vi "PrefDialog.vi"(8 "error in (no error)":errorcluster, 11 "MyPluginsBase in":refnum<class "ChromaAcLoad.lvclass">) -> (0 "error out":errorcluster, 1 "Save As":bool, 2 "Changed":bool, 3 "MyPluginsBase out":refnum<class "ChromaAcLoad.lvclass">)   [LabVIEW 2018, in "AcPwrPlugins.lvlib" / "ChromaAcLoad.lvclass"]
doc: "This VI opens up the modal preference dialog window and allows a user to configure the dialog with a new configuration or the existing configuration that was previously saved to file. The user can also chose to save the new configuration to the existing file location with the save boolean or a new file location by using the save as boolean."
uses:
  ChromaAcLoad.lvclass
  C:/Program Files (x86)/National Instruments/LabVIEW 2018/user.lib/NIST/BaseClasses/BasePlugin_class/BasePlugin.lvclass
  C:/Users/ico/Documents/Projects/NistPluggableModules/AcPwr/AcPwrPlugins/AcPwrBaseClass/AcPwrBase.lvclass
  TypeDefs/Load.ctl
  TypeDefs/LoadSettings.ctl
  TypeDefs/LC.ctl
  TypeDefs/LoadModes.ctl
  AcPwrBaseClass/TypeDefs/BaseMeasure.ctl
  AcPwrBaseClass/TypeDefs/MeasType.ctl
  AcPwrBaseClass/TypeDefs/BaseConfig.ctl
  AcPwrBaseClass/TypeDefs/Phase.ctl
  <userlib>/NIST/BaseClasses/BasePlugin_class/BasePlugin.lvclass/BasePlugin.ctl
  AcPwrBaseClass/AcPwrBase.lvclass/AcPwrBase.ctl
  ChromaAcLoad.lvclass/ChromaAcLoad.ctl
  <userlib>/NIST/BaseClasses/BasePlugin_class/Accessors/Read PluginIniFilePath.vi
  AcPwrBaseClass/Accessors/Read BaseConfig.vi
  Accessors/Read Loads.vi
  AcPwrBaseClass/Accessors/Read BaseMeasures.vi
  AcPwrBaseClass/Accessors/Read RefreshTime.vi
  AcPwrBaseClass/Accessors/Write BaseConfig.vi
  Accessors/Write Loads.vi
  AcPwrBaseClass/Accessors/Write BaseMeasures.vi
  AcPwrBaseClass/Accessors/Write RefreshTime.vi
  <vilib>/Utility/config.llb/NI_LVConfig.lvlib
  AcPwrBaseClass/AcPwrBase.lvclass
panel:
  in  "Load Numerical Configuration":T1(array[cluster])
  in  "Loads":T2(array[ring])
  in  "Slew Rate (Units/S)":T3
  in  "btnSaveAs":bool
  in  "BaseConfig":T4
  in  "RefreshTime":dbl
  in  "Measurements":T6[](array[typedef])
  in  "Loads":T8[](array[typedef])
  in  "btnSave":bool
  in  "btnCancel":bool
  # "AC is compatible with: CC, CR, CP, RLC, RLC CP, and Inrush\n\nDC is compatible with: CC, CR, CP, CV, and Rectified"
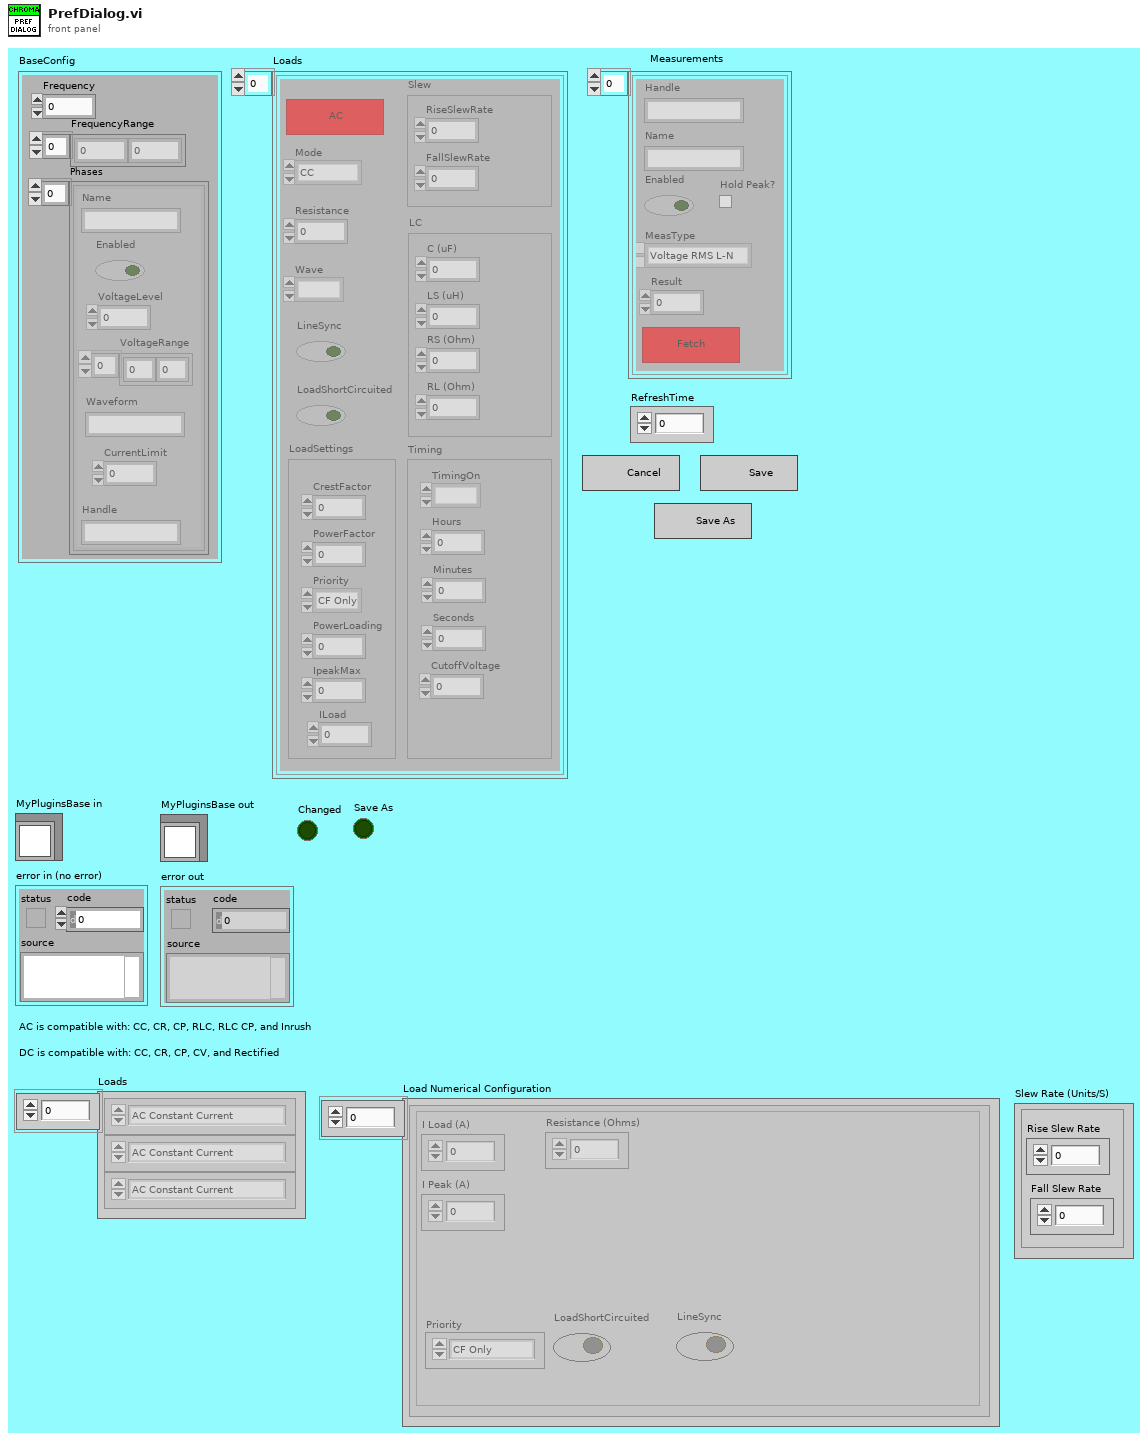
[diagram p1: front panel]
types:
  T1 = cluster{"I Load (A)":dbl, "I Peak (A)":dbl, "Resistance (Ohms)":dbl, "Priority":enum16{"CF Only", "PF Only", "Both (CF)", "Both (PF)"}, "LoadShortCircuited":bool, "LineSync":bool}[]
  T2 = enum16{"AC Constant Current", "AC Constant Resistance", "AC Constant Power", "AC RLC", "AC RL Constant Power", "AC Inrush", "DC Constant Current", "DC Constant Resistance", "DC Constant Power", "DC Constant Voltage", "DC Rectified"}[]
  T3 = cluster{"Rise Slew Rate":dbl, "Fall Slew Rate":dbl}
  T4 = typedef "AcPwrPlugins.lvlib/AcPwrBase.lvclass/BaseConfig.ctl" = cluster{"Frequency":dbl, "FrequencyRange":dbl[], "Phases":T5[]}
  T5 = typedef "AcPwrPlugins.lvlib/AcPwrBase.lvclass/Phase.ctl" = cluster{"Enabled":bool, "VoltageLevel":dbl, "Waveform":string, "Name":string, "VoltageRange":dbl[], "CurrentLimit":dbl, "Handle":string, "Connected":bool}
  T6 = typedef "AcPwrPlugins.lvlib/AcPwrBase.lvclass/BaseMeasure.ctl" = cluster{"Handle":string, "Name":string, "Enabled":bool, "Result":dbl, "MeasType":T7, "btnMeasFetch":bool, "Hold Peak?":bool}
  T7 = typedef "AcPwrPlugins.lvlib/AcPwrBase.lvclass/MeasType.ctl" = enum16{"Voltage RMS L-N", "Current RMS", "Frequency", "Voltage DC", "Current DC", "Power Factor", "Current Peak", "Power VA", "Real Power", "Voltage THD", "Voltage EHD", "Voltage OHD", "Current THD", "Current EHD", "Current OHD", "Voltage RMS L-L", "Phase Angle", "Power DC", "Crest Factor"}
  T8 = typedef "AcPwrPlugins.lvlib/ChromaAcLoad.lvclass/Load.ctl" = cluster{"AC/DC":bool, "Resistance":dbl, "LoadSettings":T9, "Wave":enum16{""}, "LineSync":bool, "LoadShortCircuited":bool, "LC":T10, "Timing":cluster{"TimingOn":enum16{""}, "Hours":u32, "Minutes":u32, "Seconds":dbl, "CutoffVoltage":dbl}, "Slew":cluster{"RiseSlewRate":i32, "FallSlewRate":i32}, "Mode":T11}
  T9 = typedef "AcPwrPlugins.lvlib/ChromaAcLoad.lvclass/LoadSettings.ctl" = cluster{"CrestFactor":dbl, "PowerFactor":dbl, "PowerLoading":dbl, "IpeakMax":dbl, "Priority":enum16{"CF Only", "PF Only", "Both (CF)", "Both (PF)"}, "ILoad":dbl}
  T10 = typedef "AcPwrPlugins.lvlib/ChromaAcLoad.lvclass/LC.ctl" = cluster{"C (uF)":i32, "LS (uH)":i32, "RL (Ohm)":dbl, "RS (Ohm)":dbl}
  T11 = typedef "AcPwrPlugins.lvlib/ChromaAcLoad.lvclass/LoadModes.ctl" = enum16{"CC", "CP", "CV", "CR", "RLC", "RLC CP", "Inrush", "Rectified"}
  T12 = enum8{"Enabled", "Disabled", "Disabled and Grayed Out"}
  T13 = enum32{"Invalid", "Default", "Floating", "Floating/Auto-Hide", "Modal"}
  T14 = enum32{"Invalid", "Standard", "Closed", "Hidden", "Minimized", "Maximized"}
  T15 = typedef "NI_LVConfig.lvlib/Config Data RefNum.ctl" = refnum<k1>
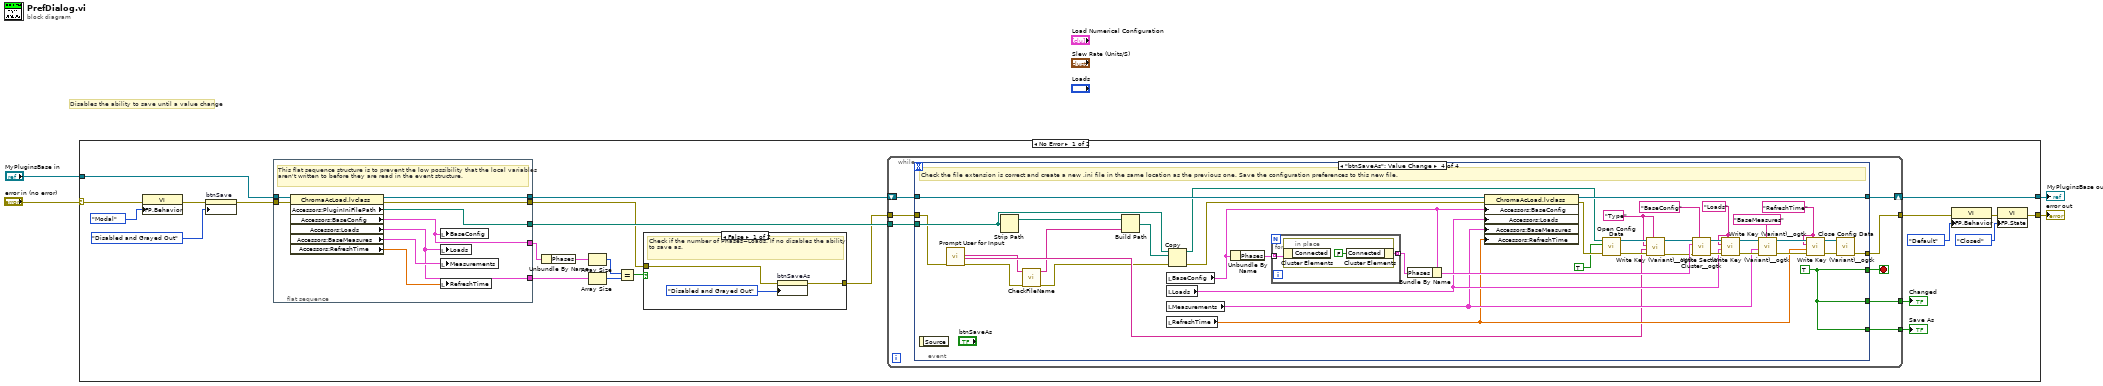
[diagram p0: block diagram]
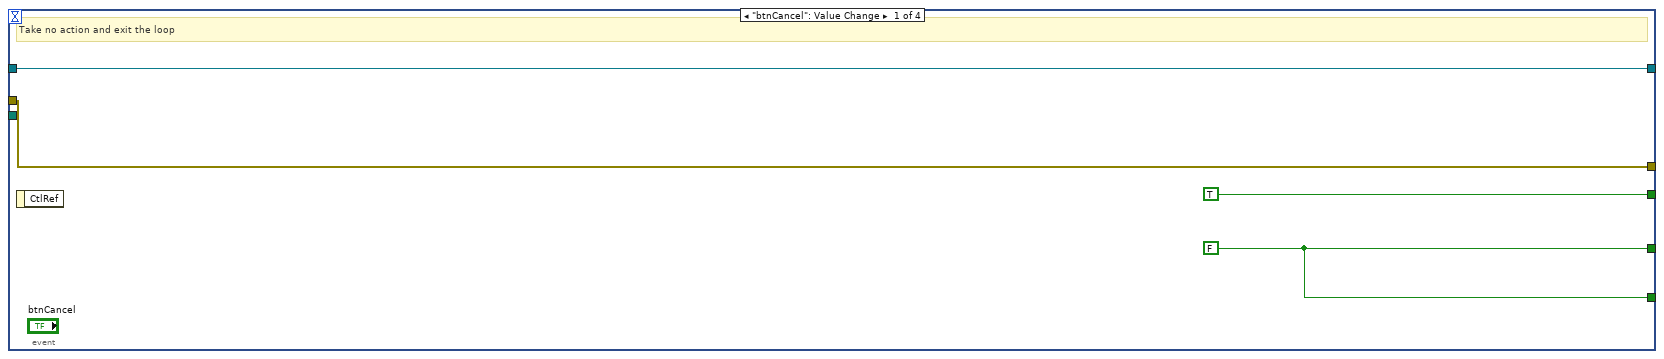
[diagram p3: hidden frame]
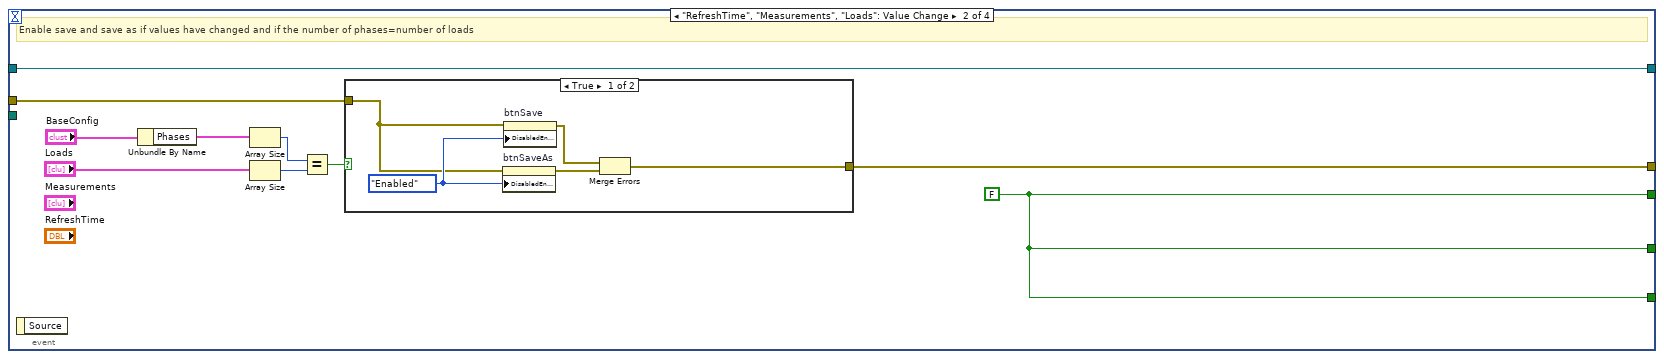
[diagram p4: hidden frame]
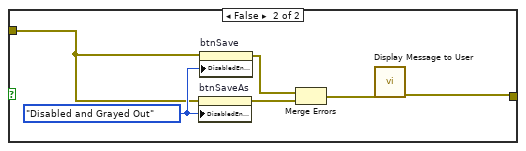
[diagram p5: hidden frame]
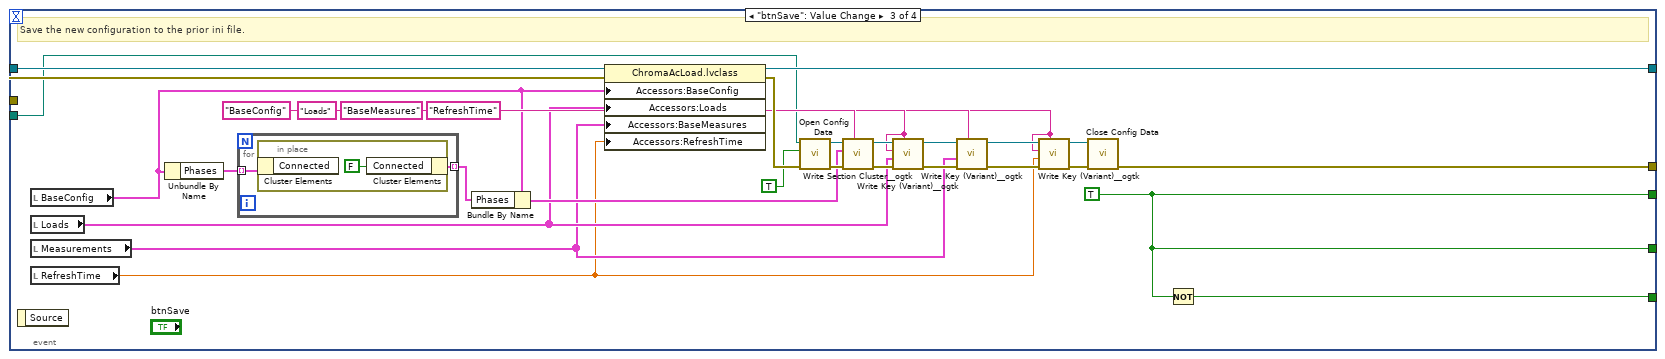
[diagram p6: hidden frame]
diagram:
  # "Disables the ability to save until a value change"
  n1 = case shown="No Error" "error in (no error)" {
    selector: "error in (no error)" -> [w19 w152]
    tunnel: [w28 w153] -> w4
    tunnel: [w24 w152] -> w3
    tunnel: "MyPluginsBase in" -> [w23 w153]
    frame No Error {
      n2 = property class="VI"(error in=w19, "FP.Behavior"=T13."Modal" ("Front Panel Window:Behavior")) -> (error out=w17:errorcluster)  [unwired: 1 in, 1 out]
      n3 = property on="btnSave" class="Bool"(error in=w17, "DisabledEnum"=T12."Disabled and Grayed Out" ("Disabled")) -> (error out=w16:errorcluster)  [unwired: 1 in, 1 out]
      n4 = flat-sequence {
        tunnel: w23 -> [w37]
        tunnel: [w36] -> w22
        tunnel: [w34] -> w9
        tunnel: w16 -> [w35]
        tunnel: [w31] -> w14
        tunnel: [w30] -> w8
        tunnel: [w29] -> w7
        frame #0 {
          # "This flat sequence structure is to prevent the low possibility that the local variables aren't written to before they are read in the event structure."
          n5 = property class="ChromaAcLoad.lvclass"(reference=w37, error in=w35) -> (reference out=w36:refnum<class "ChromaAcLoad.lvclass">, error out=w34:errorcluster, "Accessors:PluginIniFilePath"=w31:path, "Accessors:BaseConfig"=w30:T4, "Accessors:Loads"=w29:T8[], "Accessors:BaseMeasures"=w33:T6[], "Accessors:RefreshTime"=w32:dbl)
          n6 = local write "BaseConfig"(w30) -> ()
          n7 = local write "Loads"(w29) -> ()
          n8 = local write "Measurements"(w33) -> ()
          n9 = local write "RefreshTime"(w32) -> ()
        }
      }
      n10 = Unbundle By Name(w8) -> ("Phases"=w11:T5[])
      n11 = Array Size(array=w11) -> (size(s)=w12:i32)
      n12 = Array Size(array=w7) -> (size(s)=w13:i32)
      n13 = Equal?(x=w12, y=w13) -> (x = y?=w6:bool)
      n14 = case shown="False" w6 {
        tunnel: w9 -> [w38 w41]
        tunnel: [w39 w41] -> w10
        frame False {
          # "Check if the number of Phases=Loads. If no disables the ability\nto save as."
          n15 = property on="btnSaveAs" class="Bool"(error in=w38, "DisabledEnum"=T12."Disabled and Grayed Out" ("Disabled")) -> (error out=w39:errorcluster)  [unwired: 1 in, 1 out]
        }
        frame True {
        }
      }
      n16 = while {
        shift-right: [w47] -> w28
        shift-left: w22 -> [w49]
        tunnel: w10 -> [w46]
        tunnel: [w45] -> w21
        tunnel: [w44] -> w20
        tunnel: w14 -> [w43]
        tunnel: [w42] -> w5
        stop <- w48 stop-if-true
        n17 = event shown="[3] \"btnSaveAs\": Value Change" {
          selector: _ -> [_ _ _ _]
          dyn-events: _ -> [_ _ _ _]
          timeout: _ -> [_ _ _ _]
          tunnel: w49 -> [w52 w63 w99 w145]
          tunnel: [TRUE w54 w76 w113] -> w48
          tunnel: [w52 w63 w86 w133] -> w47
          tunnel: w46 -> [w51 w56 w95 w121]
          tunnel: [w51 w55 w85 w132] -> w45
          tunnel: [w50 w54 w76 w113] -> w44
          tunnel: w43 -> [_ _ w81 w123]
          tunnel: [w50 w54 w75 w113] -> w42
          event "btnCancel": Value Change {
            w50 = FALSE ("StartMeas")
            # "Take no action and exit the loop"
            n18 = event-data() -> ()  [unwired: 1 in, 1 out]
          }
          event "RefreshTime", "Measurements", "Loads": Value Change {
            w54 = FALSE
            # "Enable save and save as if values have changed and if the number of phases=number of loads"
            n19 = event-data() -> ()  [unwired: 1 in, 1 out]
            n20 = Unbundle By Name("BaseConfig") -> ("Phases"=w62:T5[])
            n21 = Array Size(array=w62) -> (size(s)=w61:i32)
            n22 = Array Size(array="Loads") -> (size(s)=w60:i32)
            n23 = Equal?(x=w61, y=w60) -> (x = y?=w59:bool)
            n24 = case shown="True" w59 {
              tunnel: w56 -> [w65 w71]
              tunnel: [w64 w69] -> w55
              frame True {
                w66 = T12."Enabled" ("Disabled")
                n25 = property on="btnSaveAs" class="Bool"(error in=w65, "DisabledEnum"=w66) -> (error out=w68:errorcluster)  [unwired: 1 in, 1 out]
                n26 = property on="btnSave" class="Bool"(error in=w65, "DisabledEnum"=w66) -> (error out=w67:errorcluster)  [unwired: 1 in, 1 out]
                n27 = Merge Errors(w67, w68) -> (w64:errorcluster)
              }
              frame False {
                w72 = T12."Disabled and Grayed Out" ("Disabled")
                n28 = property on="btnSaveAs" class="Bool"(error in=w71, "DisabledEnum"=w72) -> (error out=w74:errorcluster)  [unwired: 1 in, 1 out]
                n29 = property on="btnSave" class="Bool"(error in=w71, "DisabledEnum"=w72) -> (error out=w73:errorcluster)  [unwired: 1 in, 1 out]
                n30 = Merge Errors(w73, w74) -> (w70:errorcluster)
                n31 = call "Display Message to User"("error in (no error)"=w70) -> ("error out"=w69:errorcluster)  [unwired: 9 in, 1 out]
              }
            }
          }
          event "btnSave": Value Change {
            w82 = "RefreshTime" ("section (optional)")
            w84 = "Loads" ("section (optional)")
            w76 = TRUE
            # "Save the new configuration to the prior ini file."
            n32 = event-data() -> ()  [unwired: 1 in, 1 out]
            n33 = local read "BaseConfig"() -> (w80:T4)
            n34 = local read "Loads"() -> (w79:T8[])
            n35 = local read "Measurements"() -> (w78:T6[])
            n36 = local read "RefreshTime"() -> (w77:dbl)
            n37 = Unbundle By Name(w80) -> ("Phases"=w98:T5[])
            n38 = for {
              tunnel: w98 -> [w106] mode=indexing
              tunnel: [w105] -> w93 mode=indexing
              n39 = in-place {
                n40 = in-place-cluster #1(w106) -> ()  [unwired: 1 out]
                n41 = in-place-cluster #1("Connected"=FALSE) -> (w105:T5)
              }
            }
            n42 = Bundle By Name(cluster=w80, "Phases"=w93) -> (w94:T4)
            n43 = property class="ChromaAcLoad.lvclass"(reference=w99, error in=w95, "Accessors:BaseConfig"=w80, "Accessors:Loads"=w79, "Accessors:BaseMeasures"=w78, "Accessors:RefreshTime"=w77) -> (reference out=w86:refnum<class "ChromaAcLoad.lvclass">, error out=w104:errorcluster)
            n44 = call <vilib>:"Open Config Data.vi"("error in (no error)"=w104, "create file if necessary (T)"=TRUE, "configuration file path"=w81) -> ("error out"=w103:errorcluster, "refnum"=w102:T15)  [unwired: 6 in, 1 out]
            n45 = call <userlib>:"Write Section Cluster__ogtk.vi"("section (optional)"="BaseConfig", "error in (no error)"=w103, "Section Formatted Cluster"=w94, "refnum"=w102) -> ("error out"=w96:errorcluster, "dup refnum"=w97:T15)  [unwired: 6 in]
            n46 = call <userlib>:"Write Key (Variant)__ogtk.vi"("section"=w84, "error in (no error)"=w96, "key-value"=w79, "key (optional)"=w84, "refnum"=w97) -> ("error out"=w91:errorcluster, "refnum out"=w92:T15)  [unwired: 5 in]
            n47 = call <userlib>:"Write Key (Variant)__ogtk.vi"("section"="BaseMeasures", "error in (no error)"=w91, "key-value"=w78, "refnum"=w92) -> ("error out"=w88:errorcluster, "refnum out"=w90:T15)  [unwired: 6 in]
            n48 = call <userlib>:"Write Key (Variant)__ogtk.vi"("section"=w82, "error in (no error)"=w88, "key-value"=w77, "key (optional)"=w82, "refnum"=w90) -> ("error out"=w87:errorcluster, "refnum out"=w89:T15)  [unwired: 5 in]
            n49 = call <vilib>:"Close Config Data.vi"("error in (no error)"=w87, "refnum"=w89) -> ("error out"=w85:errorcluster)  [unwired: 8 in, 1 out]
            n50 = Not(x=w76) -> (.not. x?=w75:bool)
          }
          event "btnSaveAs": Value Change {
            w114 = "Type" ("section (optional)")
            w129 = "RefreshTime" ("section (optional)")
            w131 = "Loads" ("section (optional)")
            w113 = TRUE
            # "Check the file extension is correct and create a new .ini file in the same location as the previous one. Save the configuration preferences to this new file."
            n51 = event-data() -> ()  [unwired: 1 in, 1 out]
            n52 = call "Prompt User for Input"("error in (no error)"=w121) -> ("File Name"=w108:string, "PluginType"=w111:string, "error out"=w112:errorcluster)  [unwired: 15 in, 1 out]
            n53 = Strip Path(path=w123) -> (stripped path=w124:path)  [unwired: 1 out]
            n54 = call "CheckFileName.vi"("Error In"=w112, "File Name in"=w108) -> ("Error Out"=w110:errorcluster, "File Name out"=w109:string)  [unwired: 8 in]
            n55 = Build Path(base path=w124, name or relative path=w109) -> (appended path=w119:path)
            n56 = local read "BaseConfig"() -> (w128:T4)
            n57 = local read "Loads"() -> (w127:T8[])
            n58 = local read "Measurements"() -> (w126:T6[])
            n59 = local read "RefreshTime"() -> (w125:dbl)
            n60 = Copy(8:w110, 10:w119, 11:w123) -> (0:w120:errorcluster, 3:w122:path)  [unwired: 2 in, 1 out]
            n61 = Unbundle By Name(w128) -> ("Phases"=w144:T5[])
            n62 = for {
              tunnel: w144 -> [w150] mode=indexing
              tunnel: [w149] -> w140 mode=indexing
              n63 = in-place {
                n64 = in-place-cluster #2(w150) -> ()  [unwired: 1 out]
                n65 = in-place-cluster #2("Connected"=FALSE) -> (w149:T5)
              }
            }
            n66 = Bundle By Name(cluster=w128, "Phases"=w140) -> (w141:T4)
            n67 = property class="ChromaAcLoad.lvclass"(reference=w145, error in=w120, "Accessors:BaseConfig"=w128, "Accessors:Loads"=w127, "Accessors:BaseMeasures"=w126, "Accessors:RefreshTime"=w125) -> (reference out=w133:refnum<class "ChromaAcLoad.lvclass">, error out=w148:errorcluster)
            n68 = call <vilib>:"Open Config Data.vi"("error in (no error)"=w148, "create file if necessary (T)"=TRUE, "configuration file path"=w122) -> ("error out"=w118:errorcluster, "refnum"=w116:T15)  [unwired: 6 in, 1 out]
            n69 = call <userlib>:"Write Key (Variant)__ogtk.vi"("section"=w114, "error in (no error)"=w118, "key-value"=w111, "key (optional)"=w114, "refnum"=w116) -> ("error out"=w117:errorcluster, "refnum out"=w115:T15)  [unwired: 5 in]
            n70 = call <userlib>:"Write Section Cluster__ogtk.vi"("section (optional)"="BaseConfig", "error in (no error)"=w117, "Section Formatted Cluster"=w141, "refnum"=w115) -> ("error out"=w142:errorcluster, "dup refnum"=w143:T15)  [unwired: 6 in]
            n71 = call <userlib>:"Write Key (Variant)__ogtk.vi"("section"=w131, "error in (no error)"=w142, "key-value"=w127, "key (optional)"=w131, "refnum"=w143) -> ("error out"=w138:errorcluster, "refnum out"=w139:T15)  [unwired: 5 in]
            n72 = call <userlib>:"Write Key (Variant)__ogtk.vi"("section"="BaseMeasures", "error in (no error)"=w138, "key-value"=w126, "refnum"=w139) -> ("error out"=w135:errorcluster, "refnum out"=w137:T15)  [unwired: 6 in]
            n73 = call <userlib>:"Write Key (Variant)__ogtk.vi"("section"=w129, "error in (no error)"=w135, "key-value"=w125, "key (optional)"=w129, "refnum"=w137) -> ("error out"=w134:errorcluster, "refnum out"=w136:T15)  [unwired: 5 in]
            n74 = call <vilib>:"Close Config Data.vi"("error in (no error)"=w134, "refnum"=w136) -> ("error out"=w132:errorcluster)  [unwired: 8 in, 1 out]
          }
        }
      }
      "Changed" <- w20
      "Save As" <- w5
      n75 = property class="VI"(error in=w21, "FP.Behavior"=T13."Default" ("Front Panel Window:Behavior")) -> (error out=w27:errorcluster)  [unwired: 1 in, 1 out]
      n76 = property class="VI"(error in=w27, "FP.State"=T14."Closed" ("Front Panel Window:State")) -> (error out=w24:errorcluster)  [unwired: 1 in, 1 out]
    }
    frame Error {
    }
  }
  "error out" <- w3
  "MyPluginsBase out" <- w4
